vi "XY Graph Clip Plot Based on Graph Boundaries v2.vi"(0 "X Array in":dbl[](array[numeric]), 4 "Y Array in":dbl[](array[numeric]), 6 "Include Xmin (T)":bool=TRUE, 7 "XScale.Minimum (-Inf)":dbl=-inf, 8 "Include Xmax (T)":bool=TRUE, 9 "XScale.Maximum (Inf)":dbl=inf, 10 "Include Ymin (T)":bool=TRUE, 11 "YScale.Minimum (-Inf)":dbl=-inf, 12 "Include Ymax (T)":bool=TRUE, 13 "YScale.Maximum (Inf)":dbl=inf) -> (14 "X Array out":dbl[](array[numeric]), 18 "Y Array out":dbl[](array[numeric]))   [LabVIEW 2021, in "XY Graph Add-Ons.lvlib"]
doc: "Removes points if they are not comprised in the provided bounds."
uses:
  XY Graph Add-Ons.lvlib
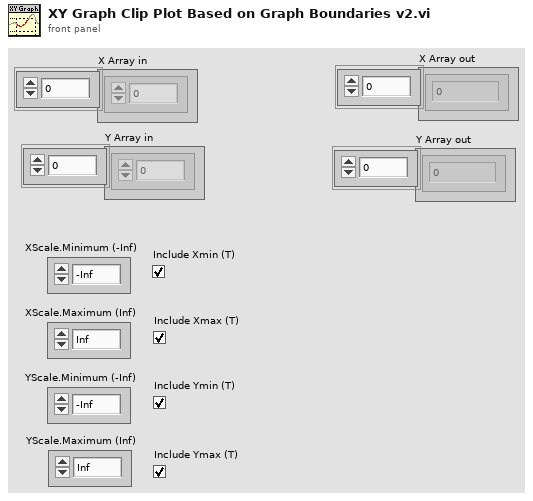
[diagram p1: front panel]
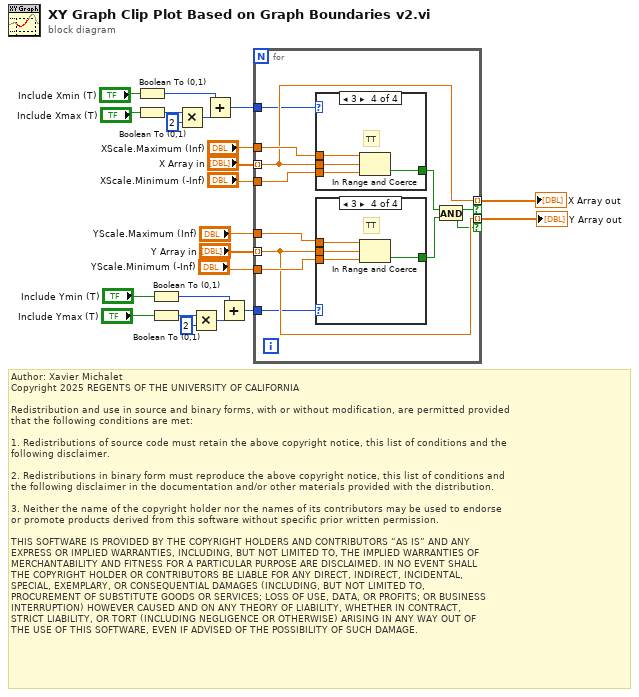
[diagram p0: block diagram]
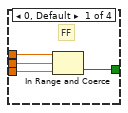
[diagram p2: hidden frame]
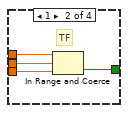
[diagram p3: hidden frame]
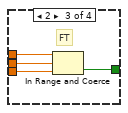
[diagram p4: hidden frame]
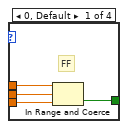
[diagram p5: hidden frame]
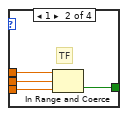
[diagram p6: hidden frame]
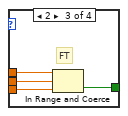
[diagram p7: hidden frame]
diagram:
  # "Author: Xavier Michalet\nCopyright 2025 REGENTS OF THE UNIVERSITY OF CALIFORNIA\n\nRedistribution and use in source and binary forms, with or without modification, are permitted provided\nthat the following conditions are met:\n\n1. Redistributions of source code must retain the above copyright notice, this list of conditions and the\nfollowing disclaimer.\n\n2. Redistributions in binary form must reproduce the above copyright notice, this list of conditions and\nthe following disclaimer in the documentation and/or other materials provided with the distribution.\n\n3. Neither the name of the copyright holder nor the names of its contributors may be used to endorse \nor promote products derived from this software without specific prior written permission.\n\nTHIS SOFTWARE IS PROVIDED BY THE COPYRIGHT HOLDERS AND CONTRIBUTORS “AS IS” AND ANY \nEXPRESS OR IMPLIED WARRANTIES, INCLUDING, BUT NOT LIMITED TO, THE IMPLIED WARRANTIES OF\nMERCHANTABILITY AND FITNESS FOR A PARTICULAR PURPOSE ARE DISCLAIMED. IN NO EVENT SHALL\nTHE COPYRIGHT HOLDER OR CONTRIBUTORS BE LIABLE FOR ANY DIRECT, INDIRECT, INCIDENTAL, \nSPECIAL, EXEMPLARY, OR CONSEQUENTIAL DAMAGES (INCLUDING, BUT NOT LIMITED TO, \nPROCUREMENT OF SUBSTITUTE GOODS OR SERVICES; LOSS OF USE, DATA, OR PROFITS; OR BUSINESS\nINTERRUPTION) HOWEVER CAUSED AND ON ANY THEORY OF LIABILITY, WHETHER IN CONTRACT, \nSTRICT LIABILITY, OR TORT (INCLUDING NEGLIGENCE OR OTHERWISE) ARISING IN ANY WAY OUT OF\nTHE USE OF THIS SOFTWARE, EVEN IF ADVISED OF THE POSSIBILITY OF SUCH DAMAGE."
  n1 = Boolean To (0,1)(Boolean="Include Xmin (T)") -> (0, 1=w12:i16)
  n2 = Boolean To (0,1)(Boolean="Include Xmax (T)") -> (0, 1=w14:i16)
  n3 = Boolean To (0,1)(Boolean="Include Ymin (T)") -> (0, 1=w8:i16)
  n4 = Boolean To (0,1)(Boolean="Include Ymax (T)") -> (0, 1=w6:i16)
  n5 = Multiply(x=w14, y=i16 2) -> (x*y=w11:i16)
  n6 = Multiply(x=w6, y=i16 2) -> (x*y=w9:i16)
  n7 = Add(x=w12, y=w11) -> (x+y=w10:i16)
  n8 = Add(x=w8, y=w9) -> (x+y=w3:i16)
  n9 = for {
    tunnel: "X Array in" -> [w31] mode=indexing
    tunnel: "Y Array in" -> [w26] mode=indexing
    tunnel: "XScale.Minimum (-Inf)" -> [w33]
    tunnel: "XScale.Maximum (Inf)" -> [w32]
    tunnel: [w31] -> w18 mode=indexing if=w23
    tunnel: "YScale.Minimum (-Inf)" -> [w28]
    tunnel: "YScale.Maximum (Inf)" -> [w27]
    tunnel: [w26] -> w17 mode=indexing if=w23
    tunnel: w10 -> [w29]
    tunnel: w3 -> [w25]
    n10 = case shown="3" w29 {
      tunnel: w33 -> [w53 w57 w61 w65]
      tunnel: w32 -> [w52 w56 w60 w64]
      tunnel: w31 -> [w51 w55 w59 w63]
      tunnel: [w50 w54 w58 w62] -> w30
      frame 0, Default {
        # "FF"
        n11 = In Range and Coerce(upper limit=w52, x=w51, lower limit=w53) -> (In Range?=w50:bool)  [unwired: 1 out]
      }
      frame 1 {
        # "TF"
        n12 = In Range and Coerce(upper limit=w56, x=w55, lower limit=w57) -> (In Range?=w54:bool)  [unwired: 1 out]
      }
      frame 2 {
        # "FT"
        n13 = In Range and Coerce(upper limit=w60, x=w59, lower limit=w61) -> (In Range?=w58:bool)  [unwired: 1 out]
      }
      frame 3 {
        # "TT"
        n14 = In Range and Coerce(upper limit=w64, x=w63, lower limit=w65) -> (In Range?=w62:bool)  [unwired: 1 out]
      }
    }
    n15 = case shown="3" w25 {
      tunnel: w28 -> [w37 w41 w45 w49]
      tunnel: w27 -> [w36 w40 w44 w48]
      tunnel: w26 -> [w35 w39 w43 w47]
      tunnel: [w34 w38 w42 w46] -> w24
      frame 0, Default {
        # "FF"
        n16 = In Range and Coerce(upper limit=w36, x=w35, lower limit=w37) -> (In Range?=w34:bool)  [unwired: 1 out]
      }
      frame 1 {
        # "TF"
        n17 = In Range and Coerce(upper limit=w40, x=w39, lower limit=w41) -> (In Range?=w38:bool)  [unwired: 1 out]
      }
      frame 2 {
        # "FT"
        n18 = In Range and Coerce(upper limit=w44, x=w43, lower limit=w45) -> (In Range?=w42:bool)  [unwired: 1 out]
      }
      frame 3 {
        # "TT"
        n19 = In Range and Coerce(upper limit=w48, x=w47, lower limit=w49) -> (In Range?=w46:bool)  [unwired: 1 out]
      }
    }
    n20 = And(x=w30, y=w24) -> (x .and. y?=w23:bool)
  }
  "X Array out" <- w18
  "Y Array out" <- w17
